vi "Create Stop Gesture.vi"() -> (3 "Gesture out":refnum<class "Gesture.lvclass">)   [LabVIEW 2023, in "Gesture.lvclass"]
uses:
  Gesture.lvclass
  Gesture Enum.ctl
  Gesture.lvclass/Gesture.ctl
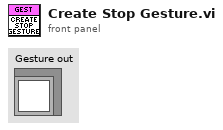
[diagram p1: front panel]
types:
  T1 = typedef "Gesture.lvclass/Gesture Enum.ctl" = enum16{"None", "Stop", "Tap", "Press", "Pan Start", "Pan Continue", "Pan End", "Pinch Open", "Pinch Close", "Double Tap"}
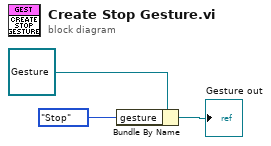
[diagram p0: block diagram]
diagram:
  n1 = Bundle By Name(cluster=refnum<class "Gesture.lvclass"> refnum ("Gesture in"), "gesture"=Gesture_Enum."Stop") -> (→"Gesture out":refnum<class "Gesture.lvclass">)
